vi "FRCts20_WebMethods_Convert_Events.vi"(8 "error in (no error)":errorcluster, 11 "EventRoot Out":T10) -> (0 "error out":errorcluster, 3 "Universe":T1)   [LabVIEW 2014, in "FRCts20_WebMethods.lvlib"]
uses:
  FRCts20_WebMethods.lvlib
  Backend/source/VI Source/FRCts20_Backend_API/FRCts20_Backend_API_EventRoot.ctl
  ESP Engine/source/VI Source/TypeDefs/FRCts20_EspEngine_Universe.ctl
  ESP Engine/source/VI Source/TypeDefs/FRCts20_EspEngine_Team.ctl
  Web Method Public Interface/FRCts20_WebMethods_ctl_singleTeam.ctl
  Web Method Public Interface/FRCts20_WebMethods_ctl_teamIdentifier.ctl
  Backend/source/VI Source/FRCts20_Backend_API/FRCts20_Backend_API_SW.ctl
  Web Method Public Interface/FRCts20_WebMethods_ctl_request.ctl
  Backend/source/VI Source/FRCts20_Backend_API/FRCts20_Backend_API_Status.ctl
  ESP Engine/source/VI Source/TypeDefs/FRCts20_EspEngine_Event.ctl
  Web Method Public Interface/FRCts20_WebMethods_ctl_singleEvent.ctl
  Backend/source/VI Source/FRCts20_Backend_API/FRCts20_Backend_API.lvlib
  ESP Engine/source/VI Source/FRCts20_EspEngine.lvlib
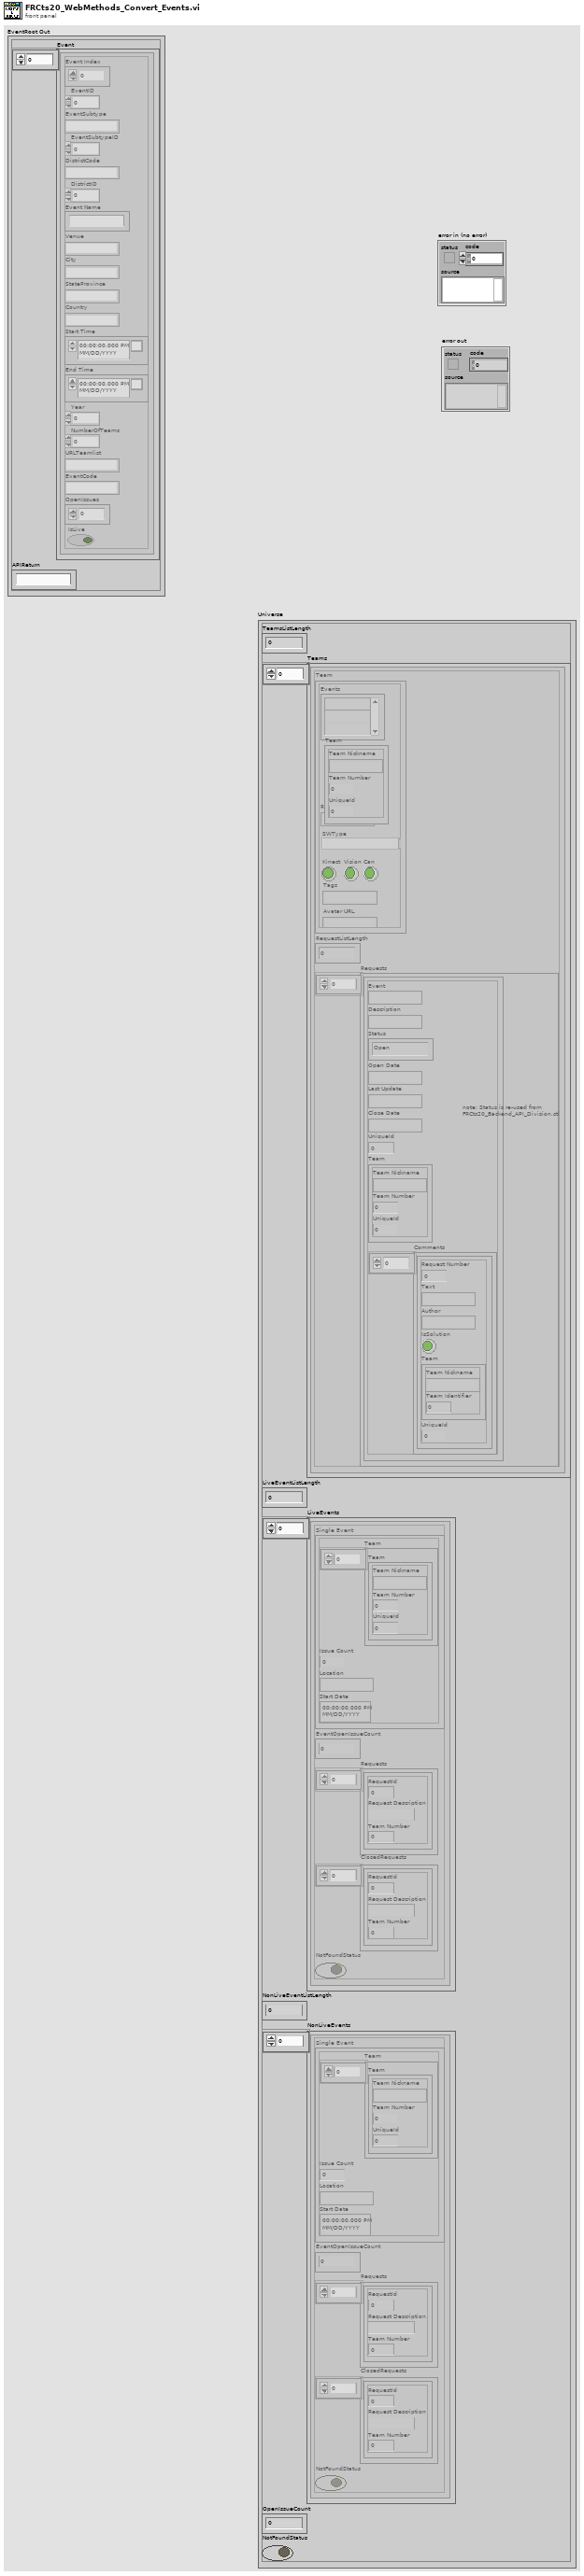
[diagram p1: front panel]
types:
  T1 = typedef "FRCts20_EspEngine.lvlib/FRCts20_EspEngine_Universe.ctl" = cluster{"TeamsListLength":i16, "Teams":T2[], "LiveEventListLength":i16, "LiveEvents":T8[], "NonLiveEventListLength":i16, "NonLiveEvents":T8[], "OpenIssueCount":i16, "NotFoundStatus":bool}
  T2 = typedef "FRCts20_EspEngine.lvlib/FRCts20_EspEngine_Team.ctl" = cluster{"Team":T3, "RequestListLength":i16, "Requests":T6[]}
  T3 = typedef "FRCts20_WebMethods.lvlib/FRCts20_WebMethods_ctl_singleTeam.ctl" = cluster{"Events":string[], "Robot Name":string, "Kinect":bool, "Vision":bool, "Can":bool, "Tags":string, "Avatar URL":string, "Team":T4, "SWType":T5}
  T4 = typedef "FRCts20_WebMethods.lvlib/FRCts20_WebMethods_ctl_teamIdentifier.ctl" = cluster{"Team Nickname":string, "Team Number ":u32, "UniqueId":u32}
  T5 = typedef "FRCts20_Backend_API.lvlib/FRCts20_Backend_API_SW.ctl" = string
  T6 = typedef "FRCts20_WebMethods.lvlib/FRCts20_WebMethods_ctl_request.ctl" = cluster{"Event":string, "Description":string, "Status":T7, "Open Date":string, "Last Update":string, "Close Date":string, "UniqueId":i32, "Team":cluster{"Team Nickname":string, "Team Number ":i32, "UniqueId":i32}, "Comments":cluster{"Request Number":dbl, "Text":string, "Author":string, "IsSolution":bool, "Team":cluster{"Team Nickname":string, "Team Identifier ":dbl}, "UniqueId":i32}[]}
  T7 = typedef "FRCts20_Backend_API.lvlib/FRCts20_Backend_API_Status.ctl" = enum16{"Open", "In Work", "Closed"}
  T8 = typedef "FRCts20_EspEngine.lvlib/FRCts20_EspEngine_Event.ctl" = cluster{"Single Event":T9, "EventOpenIssueCount":i16, "Requests":cluster{"RequestId":i32, "Request Description":string, "Team Number":i32}[], "ClosedRequests":cluster{"RequestId":i32, "Request Description":string, "Team Number":i32}[], "NotFoundStatus":bool}
  T9 = typedef "FRCts20_WebMethods.lvlib/FRCts20_WebMethods_ctl_singleEvent.ctl" = cluster{"Team":T4[], "Issue Count":i32, "Location":string, "Start Date ":timestamp}
  T10 = typedef "FRCts20_Backend_API.lvlib/FRCts20_Backend_API_EventRoot.ctl" = cluster{"Event":cluster{"Event Index":u32, "EventID":u32, "EventSubtype":string, "EventSubtypeID":u32, "DistrictCode":string, "DistrictID":u32, "Event Name":string, "Venue":string, "City":string, "StateProvince":string, "Country":string, "Start Time":timestamp, "End Time":timestamp, "Year":u32, "NumberOfTeams":u32, "URLTeamlist":string, "EventCode":string, "OpenIssues":u8, "IsLive":bool}[], "APIReturn":string}
  T11 = cluster{"Event Index":u32, "EventID":u32, "EventSubtype":string, "EventSubtypeID":u32, "DistrictCode":string, "DistrictID":u32, "Event Name":string, "Venue":string, "City":string, "StateProvince":string, "Country":string, "Start Time":timestamp, "End Time":timestamp, "Year":u32, "NumberOfTeams":u32, "URLTeamlist":string, "EventCode":string, "OpenIssues":u8, "IsLive":bool}[]
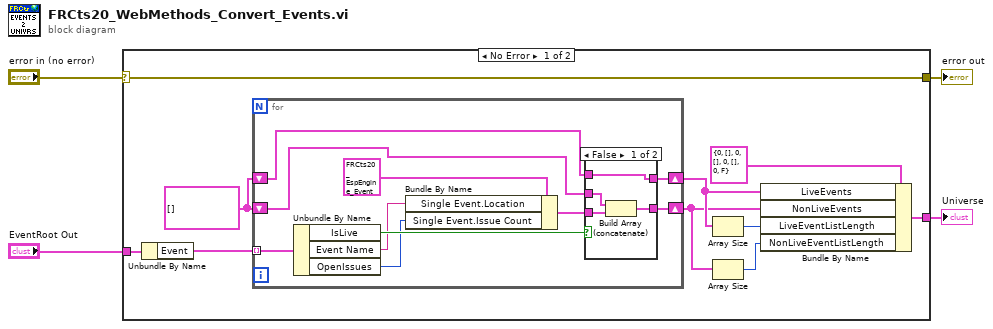
[diagram p0: block diagram]
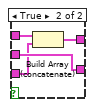
[diagram p2: hidden frame]
diagram:
  n1 = case shown="No Error" "error in (no error)" {
    selector: "error in (no error)" -> [w11 w33]
    tunnel: [w11 w33] -> w4
    tunnel: "EventRoot Out" -> [w12 _]
    tunnel: [w9 _] -> w1
    frame No Error {
      w13 = T8[] [] ("Live Events")
      n2 = Unbundle By Name(w12) -> ("Event"=w14:T11)
      n3 = for {
        tunnel: w14 -> [w24] mode=indexing
        shift-right: [w21] -> w8
        shift-left: w13 -> [w23]
        shift-right: [w20] -> w6
        shift-left: w13 -> [w22]
        n4 = Unbundle By Name(w24) -> ("IsLive"=w19:bool, "Event Name"=w17:string, "OpenIssues"=w16:u8)
        n5 = Bundle By Name(cluster=T8 {"Single Event"={"Team"=[], "Issue Count"=0, "Location"="", "Start Date "=timestamp(0 s since 1904-01-01)}, "EventOpenIssueCount"=0, "Requests"=[], "ClosedRequests"=[], "NotFoundStatus"=FALSE} ("Event"), "Single Event.Location"=w17, "Single Event.Issue Count"=w16) -> (w15:T8)
        n6 = case shown="False" w19 {
          tunnel: w22 -> [w28 w30]
          tunnel: w23 -> [w26 w32]
          tunnel: [w26 w31] -> w21
          tunnel: [w27 w30] -> w20
          tunnel: w15 -> [w25 w29]
          frame False {
            n7 = Build Array (concatenate)(w28, w25) -> (w27:T8[])
          }
          frame True {
            n8 = Build Array (concatenate)(w32, w29) -> (w31:T8[])
          }
        }
      }
      n9 = Array Size(array=w8) -> (size(s)=w7:i32)
      n10 = Array Size(array=w6) -> (size(s)=w5:i32)
      n11 = Bundle By Name(cluster=T1 {"TeamsListLength"=0, "Teams"=[], "LiveEventListLength"=0, "LiveEvents"=[], "NonLiveEventListLength"=0, "NonLiveEvents"=[], "OpenIssueCount"=0, "NotFoundStatus"=FALSE} ("Universe"), "LiveEvents"=w8, "NonLiveEvents"=w6, "LiveEventListLength"=w7, "NonLiveEventListLength"=w5) -> (w9:T1)
    }
    frame Error {
    }
  }
  "error out" <- w4
  "Universe" <- w1
